vi "例4.6 带条件端子的For循环.vi"() -> ()   [LabVIEW 2017]
panel:
  out "数值 2":dbl
  out "数值":dbl
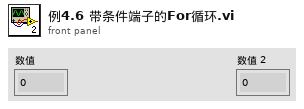
[diagram p1: front panel]
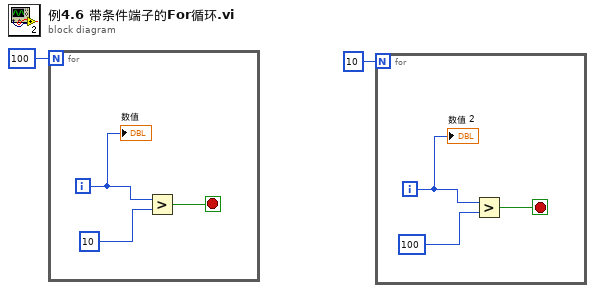
[diagram p0: block diagram]
diagram:
  n1 = for {
    N: 100 -> [_]
    i -> [w5]
    stop <- w3 stop-if-true
    n2 = Greater?(x=w5, y=10) -> (0:w3:bool)
    "数值" <- w5
  }
  n3 = for {
    N: 10 -> [_]
    i -> [w8]
    stop <- w6 stop-if-true
    n4 = Greater?(x=w8, y=100) -> (0:w6:bool)
    "数值 2" <- w8
  }
